vi "ZCAN_Receive_Data.vi"(9 "can_handle":u32) -> (0 "error out":errorcluster caption="错误输出", 1 "status":bool, 2 "CAN FDDATA":string, 3 "CAN DATA":string)   [LabVIEW 2020, in "zlgcan.lvlib"]
uses:
  zlgcan.lvlib
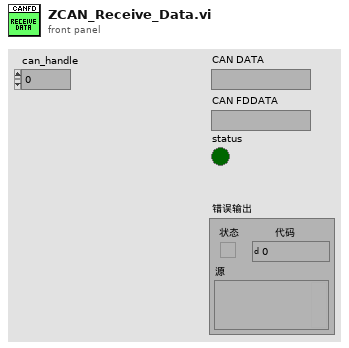
[diagram p1: front panel]
types:
  T1 = cluster{u32, u8, u8, u8, u8, cluster{"[0]":u8, "[1]":u8, "[2]":u8, "[3]":u8, "[4]":u8, "[5]":u8, "[6]":u8, "[7]":u8, "[8]":u8, "[9]":u8, "[10]":u8, "[11]":u8, "[12]":u8, "[13]":u8, "[14]":u8, "[15]":u8, "[16]":u8, "[17]":u8, "[18]":u8, "[19]":u8, "[20]":u8, "[21]":u8, "[22]":u8, "[23]":u8, "[24]":u8, "[25]":u8, "[26]":u8, "[27]":u8, "[28]":u8, "[29]":u8, "[30]":u8, "[31]":u8, "[32]":u8, "[33]":u8, "[34]":u8, "[35]":u8, "[36]":u8, "[37]":u8, "[38]":u8, "[39]":u8, "[40]":u8, "[41]":u8, "[42]":u8, "[43]":u8, "[44]":u8, "[45]":u8, "[46]":u8, "[47]":u8, "[48]":u8, "[49]":u8, "[50]":u8, "[51]":u8, "[52]":u8, "[53]":u8, "[54]":u8, "[55]":u8, "[56]":u8, "[57]":u8, "[58]":u8, "[59]":u8, "[60]":u8, "[61]":u8, "[62]":u8, "[63]":u8}, u64}[]
  T2 = cluster{u32, u8, u8, u8, u8, cluster{"[0]":u8, "[1]":u8, "[2]":u8, "[3]":u8, "[4]":u8, "[5]":u8, "[6]":u8, "[7]":u8}, u64}[]
  T3 = cluster{"[0]":u8, "[1]":u8, "[2]":u8, "[3]":u8, "[4]":u8, "[5]":u8, "[6]":u8, "[7]":u8}
  T4 = cluster{"[0]":u8, "[1]":u8, "[2]":u8, "[3]":u8, "[4]":u8, "[5]":u8, "[6]":u8, "[7]":u8, "[8]":u8, "[9]":u8, "[10]":u8, "[11]":u8, "[12]":u8, "[13]":u8, "[14]":u8, "[15]":u8, "[16]":u8, "[17]":u8, "[18]":u8, "[19]":u8, "[20]":u8, "[21]":u8, "[22]":u8, "[23]":u8, "[24]":u8, "[25]":u8, "[26]":u8, "[27]":u8, "[28]":u8, "[29]":u8, "[30]":u8, "[31]":u8, "[32]":u8, "[33]":u8, "[34]":u8, "[35]":u8, "[36]":u8, "[37]":u8, "[38]":u8, "[39]":u8, "[40]":u8, "[41]":u8, "[42]":u8, "[43]":u8, "[44]":u8, "[45]":u8, "[46]":u8, "[47]":u8, "[48]":u8, "[49]":u8, "[50]":u8, "[51]":u8, "[52]":u8, "[53]":u8, "[54]":u8, "[55]":u8, "[56]":u8, "[57]":u8, "[58]":u8, "[59]":u8, "[60]":u8, "[61]":u8, "[62]":u8, "[63]":u8}
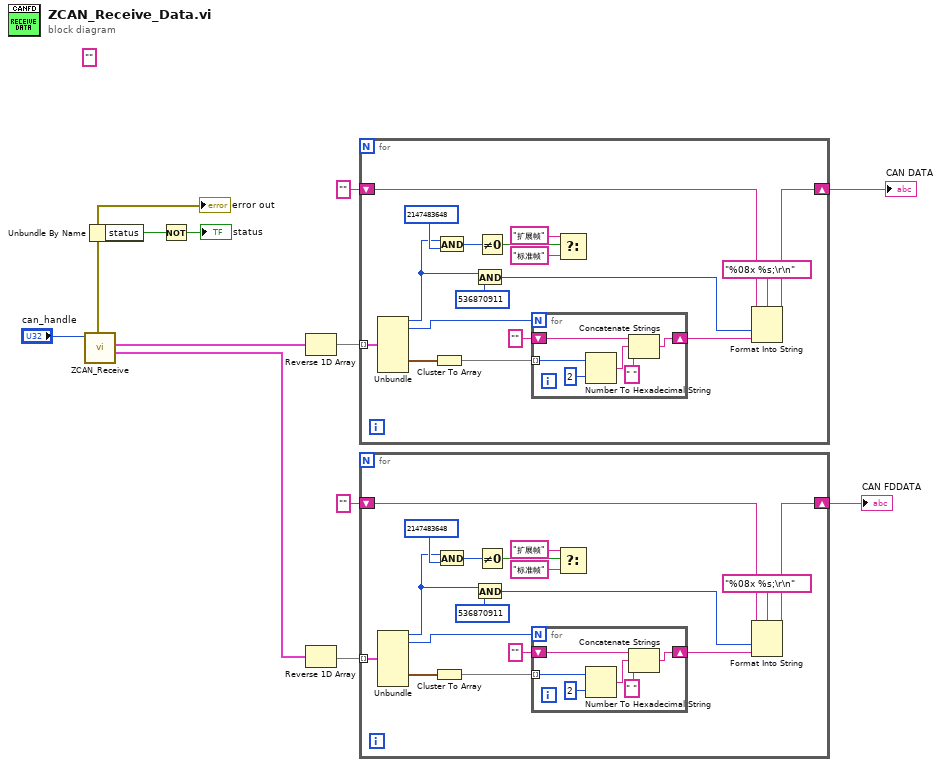
[diagram p0: block diagram]
diagram:
  (unwired) ""
  n1 = call "ZCAN_Receive.vi"("can_handle"="can_handle") -> ("error out"=w11:errorcluster, "CANFD数据帧数组"=w7:T1, "CAN数据帧数组"=w8:T2)  [unwired: 3 in, 1 out]
  "error out" <- w11
  n2 = Unbundle By Name(w11) -> ("status"=w10:bool)
  n3 = Not(x=w10) -> (.not. x?=→"status":bool)
  n4 = Reverse 1D Array(array=w8) -> (reversed array=w6:T2)
  n5 = Reverse 1D Array(array=w7) -> (reversed array=w2:T1)
  n6 = for {
    tunnel: w6 -> [w29] mode=indexing
    shift-right: [w14] -> w4
    shift-left: "" -> [w13]
    n7 = Unbundle(w29) -> (w19:u32, w18:u8, w22:T3)  [unwired: 4 out]
    n8 = Cluster To Array(cluster=w22) -> (array=w21:u8[])
    n9 = And(x=w19, y=u32 2147483648) -> (x .and. y?=w27:u32)
    n10 = And(x=w19, y=u32 536870911) -> (x .and. y?=w17:u32)
    n11 = Not Equal To 0?(x=w27) -> (x != 0?=w26:bool)
    n12 = for {
      N: w18 -> [_]
      shift-right: [w32] -> w16
      shift-left: "" -> [w30]
      tunnel: w21 -> [w31] mode=indexing
      n13 = Number To Hexadecimal String(1:i16 2 ("width (-)"), 2:w31) -> (0:w34:string)
      n14 = Concatenate Strings(w30, w34, " " ("string")) -> (w32:string)
    }
    n15 = Select(t="扩展帧", s=w26, f="标准帧") -> ()  [unwired: 1 out]
    n16 = Format Into String(format string="%08x %s;\r\n", initial string=w13, w17, w16) -> (resulting string=w14:string)  [unwired: 1 in, 1 out]
  }
  "CAN DATA" <- w4
  n17 = for {
    tunnel: w2 -> [w52] mode=indexing
    shift-right: [w37] -> w1
    shift-left: "" -> [w36]
    n18 = Unbundle(w52) -> (w42:u32, w41:u8, w45:T4)  [unwired: 4 out]
    n19 = Cluster To Array(cluster=w45) -> (array=w44:u8[])
    n20 = And(x=w42, y=u32 2147483648) -> (x .and. y?=w50:u32)
    n21 = And(x=w42, y=u32 536870911) -> (x .and. y?=w40:u32)
    n22 = Not Equal To 0?(x=w50) -> (x != 0?=w49:bool)
    n23 = for {
      N: w41 -> [_]
      shift-right: [w55] -> w39
      shift-left: "" -> [w53]
      tunnel: w44 -> [w54] mode=indexing
      n24 = Number To Hexadecimal String(1:i16 2 ("width (-)"), 2:w54) -> (0:w57:string)
      n25 = Concatenate Strings(w53, w57, " " ("string")) -> (w55:string)
    }
    n26 = Select(t="扩展帧", s=w49, f="标准帧") -> ()  [unwired: 1 out]
    n27 = Format Into String(format string="%08x %s;\r\n", initial string=w36, w40, w39) -> (resulting string=w37:string)  [unwired: 1 in, 1 out]
  }
  "CAN FDDATA" <- w1
